vi "FRC Color Processing.vi"() -> ()   [LabVIEW 2017]
uses:
  <vilib>/Rock Robotics/WPI/Camera/WPI_CameraSettings Read MJPG.ctl
  <vilib>/Rock Robotics/WPI/Camera/WPI_CameraImageSize.ctl
  Vision Support Code/Camera Types.ctl
  <vilib>/Rock Robotics/WPI/Camera/WPI_CameraExposure Values.ctl
  <vilib>/Rock Robotics/WPI/Camera/WPI_CameraWhite Balance Values.ctl
  <vilib>/Rock Robotics/WPI/DriverStation/WPI_DriverStationAllianceInfo.ctl
  <vilib>/vision/NI_Vision_Development_Module.lvlib
panel:
  in  "Ring":u16(ring) items=["Cube", "Tape", "Switch LED", "Scale LED"]
  out "Angles":cluster{"Azimuth":dbl, "Elevation":dbl}[](array[cluster])
  in  "Vision Color Mode":u16(ring) items=["Alliance Color Range", "Reflective Tape", "Manual Color Range"]
  out "Game Specific Data":string
  out "Alliance":T1
  in  "Camera Address":string="USB 0"
  in  "Camera Settings":T2={"fps"=20, "compression"=30, "Image Size"=enum."320x240", "Config Shown"=FALSE}
  in  "Camera Settings 2":T6={"Exposure"=enum."Auto", "Exposure (%)"=50.0, "Brightness"=50, "White Balance"=enum."Auto", "Color Temp (K)"=0.0} {"Brightness" min=0 max=100}
  in  "Min Compnt %":dbl=15.0
  out "Results":T7(array[cluster]) {"Score" format="%#_3g"; "Pixels"."Rectangle"."Numeric 5" format="%#_3g"; "Pixels"."Rectangle"."Numeric 3" format="%#_3g"; "Pixels"."Rectangle"."Numeric 2" format="%#_3g"; "Pixels"."Rectangle"."Numeric" format="%#_3g"; "Normalized"."Rectangle"."Numeric 5" format="%#_2g"; "Normalized"."Rectangle"."Numeric 3" format="%#_2g"; "Normalized"."Rectangle"."Numeric 2" format="%#_2g"; "Normalized"."Rectangle"."Numeric" format="%#_2g"; "Normalized"."Center"."?" format="%#_3g"; "Normalized"."Center"."?" format="%#_3g"; "Distance (ft)" format="%#_3g"}
  in  "Size Limit %":dbl=0.04 min=0.0 max=100.0 step=0.01 format="%#_13g"
  out "Instructions:":string="Instructions:\nUse Source to load image files from a directory, or use a USB or IP camera connected to your laptop. Use Camera Settings 1 and 2 to achieve a dark image with bright and colorful stripes.\nLED Color can encoded as HSL or related color modes. Calibrate to the same color as the strips being reflected to the camera.\nClick and draw a line in Original Image to auto-calibrate the LED Color. You may want to widen and tweak Sat and Val by hand.\nThe Annotate button affects drawing a rectangle around the stripes and labeling it with a distance in ft. Distance relies on knowing the Camera Type and lens calibration (it looks up the lens view angle).\n\nAdjust Score Cutoff to make the code more or less picky. If the color is not very unique, you may need to increase the number of particles considered. The diagram uses a Size Limit to ignore colored things that are too small. You may need to adjust it if you are targetting from far away.\n\nResults give you the distance to the target, the center and box in a normalized (-1 to 1) and pixel coordinates.\n\nBe sure to read about setting camera exposure and brightness to help simplify your image and acquire color saturated images.\n\nThere are lots of comments on the diagram to explain the code."
  in  "Color Mode":u16(ring)=2 items=["RGB", "HSL", "HSV", "HSI"]
  in  "Particles":dbl=5.0
  in  "Score Cutoff %":dbl=75.0
  in  "Std Devs for Calibration":cluster{"H":dbl, "S":dbl, "V":dbl}={"H"=4.0, "S"=8.0, "V"=8.0}
  in  "Camera Type (for distance)":T8=enum."MS HD3000 square"
  in  "Annotate":bool=TRUE
  out "Qualified Particles":i32
  in  "LED Color Range":T9={"Hue"={75.46666717529297, 107.46666717529297}, "Sat"={221.18788146972656, 255.0}, "Val"={23.733230590820312, 172.13343811035156}} {"Hue" scale=0.0..255.0 scale format="%#_3g"}
  out "Mask":T10(plugin-control)
  out "Original Image":T10(plugin-control)
  # "Good target rectangle, distance ft"
  # "Bad target rectangle"
  # "Score in %"
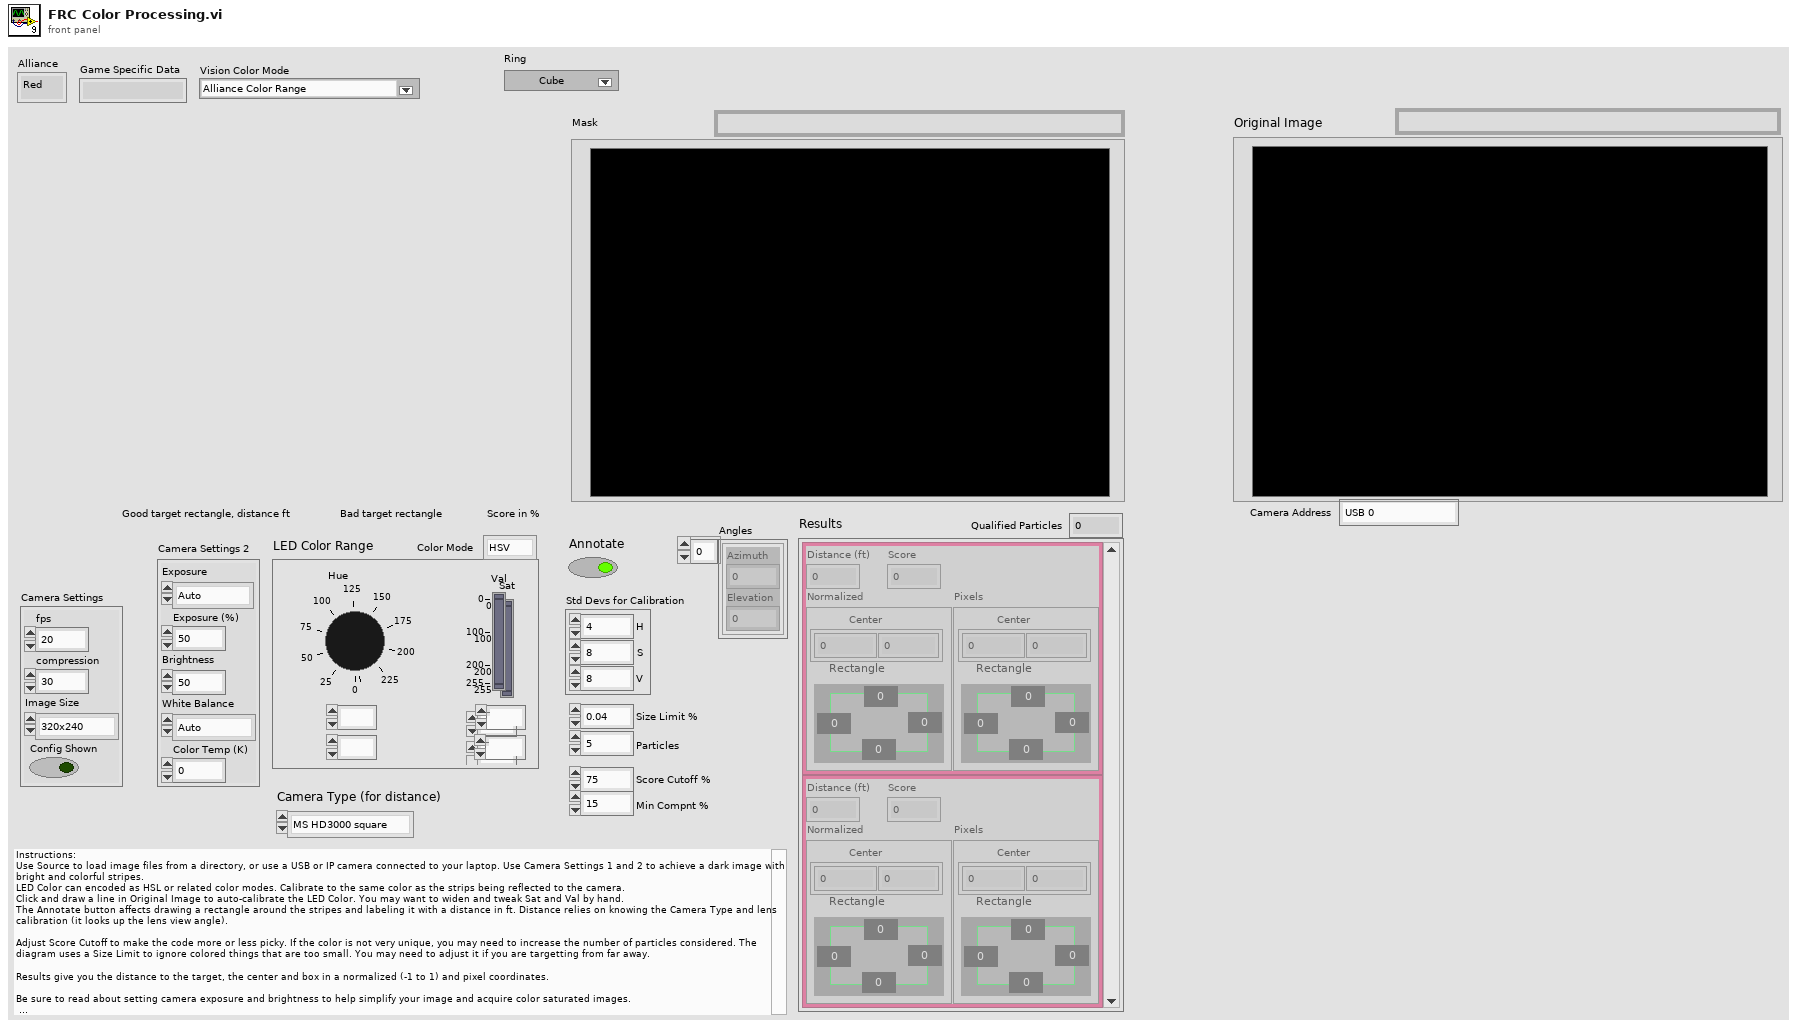
[diagram p1: front panel]
types:
  T1 = typedef "WPI_DriverStationAllianceInfo.ctl" = enum16{"Red", "Blue", "Invalid"}
  T2 = typedef "WPI_CameraSettings Read MJPG.ctl" = cluster{"fps":i32, "compression":i32, "Image Size":T3, "Config Shown":bool}
  T3 = typedef "WPI_CameraImageSize.ctl" = enum16{"640x480", "320x240", "160x120", "Custom"}
  T4 = typedef "WPI_CameraExposure Values.ctl" = enum16{"Auto", "Flicker-free 50 Hz", "Flicker-free 60 Hz", "Hold current", "Custom"}
  T5 = typedef "WPI_CameraWhite Balance Values.ctl" = enum16{"Auto", "Fixed indoor", "Fixed outdoor 1", "Fixed outdoor 2", "Fixed fluorescent 1", "Fixed fluorescent 2", "Hold current", "Custom"}
  T6 = cluster{"Exposure":T4, "Exposure (%)":dbl, "Brightness":i32, "White Balance":T5, "Color Temp (K)":dbl}
  T7 = cluster{"Distance (ft)":dbl, "Score":dbl, "Normalized":cluster{"Center":cluster{dbl, dbl}, "Rectangle":cluster{"Numeric":dbl, "Numeric 2":dbl, "Numeric 3":dbl, "Numeric 5":dbl}}, "Pixels":cluster{"Center":cluster{dbl, dbl}, "Rectangle":cluster{"Numeric":dbl, "Numeric 2":dbl, "Numeric 3":dbl, "Numeric 5":dbl}}}[]
  T8 = typedef "Camera Types.ctl" = enum16{"206", "1011", "1013", "MS HD3000 square", "MS HD3000 640x480"}
  T9 = cluster{"Hue":cluster{dbl, dbl}, "Sat":cluster{dbl, dbl}, "Val":cluster{dbl, dbl}}
  T10 = typedef "IMAQ Image.ctl" = refnum<image>
  T11 = typedef "Particle Parameters" = i32
  T12 = typedef "Image Type" = u32
  T13 = enum8{"Enabled", "Disabled", "Disabled and Grayed Out"}
  T14 = cluster{cluster{dbl, dbl}, cluster{dbl, dbl}, cluster{dbl, dbl}}
  T15 = cluster{"Score":dbl, "Rect":cluster{"Left":dbl, "Top":dbl, "Right":dbl, "Bottom":dbl}, "Full Scores":cluster{"Aspect Ratio":dbl, "Top Position":dbl, "Bottom Position":dbl, "Left Gap":dbl, "Width":dbl, "Height Ratio":dbl}}[]
  T16 = cluster{"Left":dbl, "Top":dbl, "Right":dbl, "Bottom":dbl}
  T17 = cluster{"Distance (ft)":dbl, "Score":dbl, "Normalized":cluster{"Center":cluster{dbl, dbl}, "Rectangle":cluster{"Numeric":dbl, "Numeric 2":dbl, "Numeric 3":dbl, "Numeric 5":dbl}}, "Pixels":cluster{"Center":cluster{dbl, dbl}, "Rectangle":cluster{"Numeric":dbl, "Numeric 2":dbl, "Numeric 3":dbl, "Numeric 5":dbl}}}
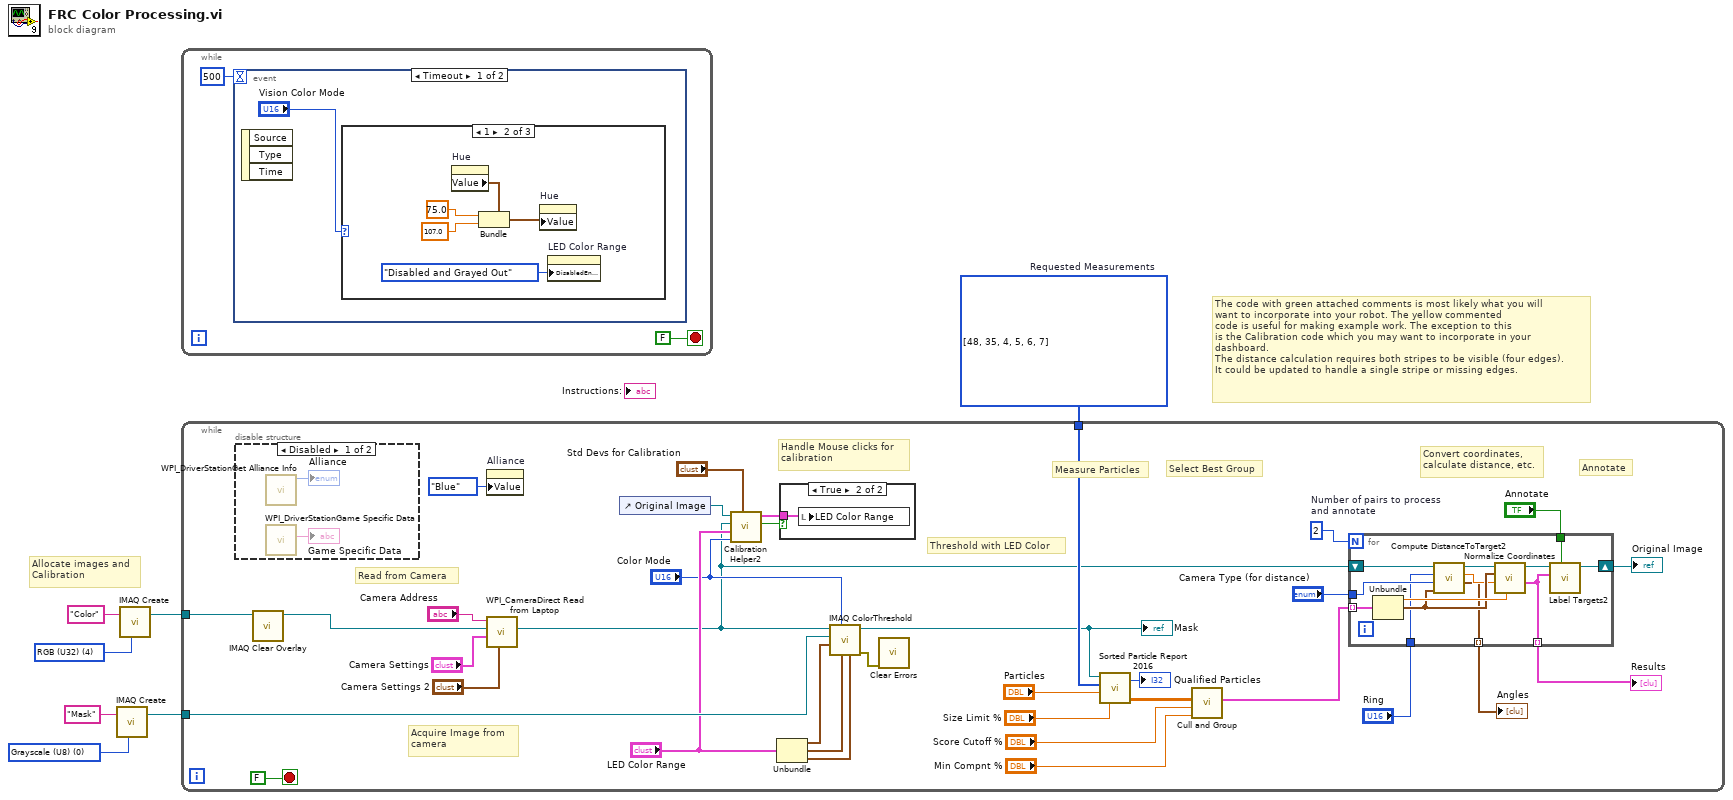
[diagram p0: block diagram]
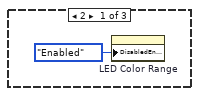
[diagram p2: hidden frame]
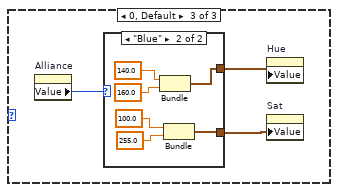
[diagram p3: hidden frame]
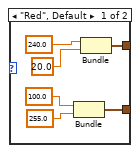
[diagram p4: hidden frame]
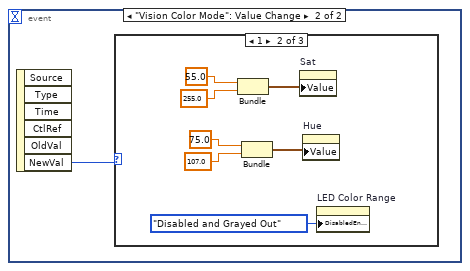
[diagram p5: hidden frame]
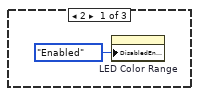
[diagram p6: hidden frame]
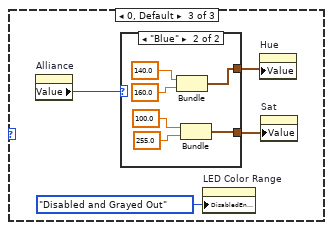
[diagram p7: hidden frame]
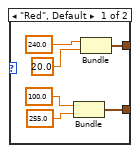
[diagram p8: hidden frame]
diagram:
  w2 = T11[] [48, 35, 4, 5, 6, 7] items=["Center of Mass X", "Center of Mass Y", "First Pixel X", "First Pixel Y", "Bounding Rect Left", "Bounding Rect Top", "Bounding Rect Right", "Bounding Rect Bottom", "Max Feret Diameter Start X", "Max Feret Diameter Start Y", "Max Feret Diameter End X", "Max Feret Diameter End Y", "Max Horiz. Segment Length Left", "Max Horiz. Segment Length Right", "Max Horiz. Segment Length Row", "-", "Bounding Rect Width", "Bounding Rect Height", "Bounding Rect Diagonal", "Perimeter", "Convex Hull Perimeter", "Holes' Perimeter", "Max Feret Diameter", "Equivalent Ellipse Major Axis", "Equivalent Ellipse Minor Axis", "Equivalent Ellipse Minor Axis (Feret)", "Equivalent Rect Long Side", "Equivalent Rect Short Side", "Equivalent Rect Diagonal", "Equivalent Rect Short Side (Feret)", "Average Horiz. Segment Length", "Average Vert. Segment Length", "Hydraulic Radius", "Waddel Disk Diameter", "-", "Area", "Holes' Area", "Particle & Holes' Area", "Convex Hull Area", "Image Area", "-", "Number of Holes", "Number of Horiz. Segments", "Number of Vert. Segments", "-", "Orientation", "Max Feret Diameter Orientation", "-", "% Area/Image Area", "% Area/(Particle & Holes' Area)", "Ratio of Equivalent Ellipse Axes", "Ratio of Equivalent Rect Sides", "-", "Elongation Factor", "Compactness Factor", "Heywood Circularity Factor", "Type Factor", "-", "Sum X", "Sum Y", "Sum XX", "Sum XY", "Sum YY", "Sum XXX", "Sum XXY", "Sum XYY", "Sum YYY", "-", "Moment of Inertia XX", "Moment of Inertia XY", "Moment of Inertia YY", "Moment of Inertia XXX", "Moment of Inertia XXY", "Moment of Inertia XYY", "Moment of Inertia YYY", "Norm. Moment of Inertia XX", "Norm. Moment of Inertia XY", "Norm. Moment of Inertia YY", "Norm. Moment of Inertia XXX", "Norm. Moment of Inertia XXY", "Norm. Moment of Inertia XYY", "Norm. Moment of Inertia YYY", "Hu Moment 1", "Hu Moment 2", "Hu Moment 3", "Hu Moment 4", "Hu Moment 5", "Hu Moment 6", "Hu Moment 7"]  # Requested Measurements
  w5 = T12 0 items=["Grayscale (U8)", "Grayscale (I16)", "Grayscale (SGL)", "Complex (CSG)", "RGB (U32)", "HSL (U32)", "RGB (U64)", "Grayscale (U16)"] ("Image Type")
  w6 = T12 4 items=["Grayscale (U8)", "Grayscale (I16)", "Grayscale (SGL)", "Complex (CSG)", "RGB (U32)", "HSL (U32)", "RGB (U64)", "Grayscale (U16)"] ("Image Type")
  # "The code with green attached comments is most likely what you will\nwant to incorporate into your robot. The yellow commented\ncode is useful for making example work. The exception to this\nis the Calibration code which you may want to incorporate in your\ndashboard.\nThe distance calculation requires both stripes to be visible (four edges).\nIt could be updated to handle a single stripe or missing edges."
  # "Allocate images and\nCalibration"
  n1 = call "IMAQ Create"("Image Name"="Mask", "Image Type"=w5) -> ("New Image"=w3:T10)  [unwired: 2 in, 2 out]
  n2 = call "IMAQ Create"("Image Name"="Color", "Image Type"=w6) -> ("New Image"=w1:T10)  [unwired: 2 in, 2 out]
  n3 = while {
    stop <- FALSE stop-if-true
    n4 = event shown="[0] Timeout" {
      selector: _ -> [_ _]
      dyn-events: _ -> [_ _]
      timeout: 500 -> [_ _]
      event Timeout {
        n5 = event-data() -> ()  [unwired: 1 in, 3 out]
        n6 = case shown="1" "Vision Color Mode" {
          frame 2 {
            n7 = property on="LED Color Range" class="Clust (strict)"("DisabledEnum"=T13."Enabled" ("Disabled")) -> ()  [unwired: 2 in, 2 out]
          }
          frame 1 {
            n8 = property on="Hue" class="Knob (strict)"() -> ("Value"=w16:cluster{dbl, dbl})  [unwired: 2 in, 2 out]
            n9 = Bundle(cluster=w16, 75.0, 107.0) -> (w15:cluster{dbl, dbl})
            n10 = property on="Hue" class="Knob (strict)"("Value"=w15) -> ()  [unwired: 2 in, 2 out]
            n11 = property on="LED Color Range" class="Clust (strict)"("DisabledEnum"=T13."Disabled and Grayed Out" ("Disabled")) -> ()  [unwired: 2 in, 2 out]
          }
          frame 0, Default {
            n12 = property on="Alliance" class="Enum (strict)"() -> ("Value"=w17:T1)  [unwired: 2 in, 2 out]
            n13 = case shown="\"Blue\"" w17 {
              tunnel: [w21 w27] -> w19
              tunnel: [w20 w26] -> w18
              frame "Red", Default {
                n14 = Bundle(100.0, 255.0) -> (w20:cluster{dbl, dbl})  [unwired: 1 in]
                n15 = Bundle(240.0, 20.0) -> (w21:cluster{dbl, dbl})  [unwired: 1 in]
              }
              frame "Blue" {
                n16 = Bundle(140.0, 160.0) -> (w27:cluster{dbl, dbl})  [unwired: 1 in]
                n17 = Bundle(100.0, 255.0) -> (w26:cluster{dbl, dbl})  [unwired: 1 in]
              }
            }
            n18 = property on="Hue" class="Knob (strict)"("Value"=w19) -> ()  [unwired: 2 in, 2 out]
            n19 = property on="Sat" class="Slide (strict)"("Value"=w18) -> ()  [unwired: 2 in, 2 out]
          }
        }
      }
      event "Vision Color Mode": Value Change {
        n20 = event-data() -> ("NewVal"=w32:u16)  [unwired: 1 in, 5 out]
        n21 = case shown="1" w32 {
          frame 2 {
            n22 = property on="LED Color Range" class="Clust (strict)"("DisabledEnum"=T13."Enabled" ("Disabled")) -> ()  [unwired: 2 in, 2 out]
          }
          frame 1 {
            n23 = Bundle(55.0, 255.0) -> (w34:cluster{dbl, dbl})  [unwired: 1 in]
            n24 = Bundle(75.0, 107.0) -> (w39:cluster{dbl, dbl})  [unwired: 1 in]
            n25 = property on="Sat" class="Slide (strict)"("Value"=w34) -> ()  [unwired: 2 in, 2 out]
            n26 = property on="Hue" class="Knob (strict)"("Value"=w39) -> ()  [unwired: 2 in, 2 out]
            n27 = property on="LED Color Range" class="Clust (strict)"("DisabledEnum"=T13."Disabled and Grayed Out" ("Disabled")) -> ()  [unwired: 2 in, 2 out]
          }
          frame 0, Default {
            n28 = property on="Alliance" class="Enum (strict)"() -> ("Value"=w41:T1)  [unwired: 2 in, 2 out]
            n29 = case shown="\"Blue\"" w41 {
              tunnel: [w46 w52] -> w43
              tunnel: [w45 w51] -> w42
              frame "Red", Default {
                n30 = Bundle(100.0, 255.0) -> (w45:cluster{dbl, dbl})  [unwired: 1 in]
                n31 = Bundle(240.0, 20.0) -> (w46:cluster{dbl, dbl})  [unwired: 1 in]
              }
              frame "Blue" {
                n32 = Bundle(140.0, 160.0) -> (w52:cluster{dbl, dbl})  [unwired: 1 in]
                n33 = Bundle(100.0, 255.0) -> (w51:cluster{dbl, dbl})  [unwired: 1 in]
              }
            }
            n34 = property on="LED Color Range" class="Clust (strict)"("DisabledEnum"=T13."Disabled and Grayed Out" ("Disabled")) -> ()  [unwired: 2 in, 2 out]
            n35 = property on="Hue" class="Knob (strict)"("Value"=w43) -> ()  [unwired: 2 in, 2 out]
            n36 = property on="Sat" class="Slide (strict)"("Value"=w42) -> ()  [unwired: 2 in, 2 out]
          }
        }
      }
    }
  }
  n37 = while {
    tunnel: w1 -> [w66]
    tunnel: w3 -> [w90]
    tunnel: w2 -> [w86]
    stop <- FALSE stop-if-true
    w68 = 2  # Number of pairs to process and annotate
    # "Read from Camera"
    # "Handle Mouse clicks for\ncalibration"
    # "Measure Particles"
    # "Convert coordinates,\ncalculate distance, etc."
    # "Annotate"
    # "Select Best Group"
    # "Threshold with LED Color"
    # "Acquire Image from\ncamera"
    n38 = disable-structure shown="Disabled" {
      frame Disabled {
        n39 = call <vilib>:"WPI_DriverStationGet Alliance Info.vi"() -> ("Alliance"=→"Alliance":T1)  [unwired: 6 in, 5 out]
        n40 = call <vilib>:"WPI_DriverStationGame Specific Data.vi"() -> ("Game Specific Data"=→"Game Specific Data":string)  [unwired: 11 in]
      }
      frame Enabled {
      }
    }
    n41 = call "IMAQ Clear Overlay"("Image"=w66) -> ("Image Out"=w65:T10)  [unwired: 2 in, 8 out]
    n42 = property on="Alliance" class="Enum (strict)"("Value"=WPI_DriverStationAllianceInfo."Blue" ("Alliance")) -> ()  [unwired: 2 in, 2 out]
    n43 = call <vilib>:"WPI_CameraDirect Read from Laptop.vi"("Camera Settings 2"="Camera Settings 2", "Camera Settings"="Camera Settings", "Image"=w65, "address"="Camera Address") -> ("Image Out"=w67:T10)  [unwired: 6 in, 1 out]
    n44 = control-ref of="Original Image"() -> (w82:refnum<vi>)
    n45 = call "Calibration Helper2.vi"("Std Devs"="Std Devs for Calibration", "Color Mode"="Color Mode", "Color Components"="LED Color Range", "Image"=w67, "Image Ctl Refnum"=w82) -> ("Changed"=w81:bool, "output color"=w80:T14)  [unwired: 5 in]
    n46 = Unbundle("LED Color Range") -> ("Hue"=w89:cluster{dbl, dbl}, "Sat"=w88:cluster{dbl, dbl}, "Val"=w87:cluster{dbl, dbl})
    n47 = case shown="True" w81 {
      tunnel: w80 -> [_ w107]
      frame False {
      }
      frame True {
        n48 = local write "LED Color Range"(w107) -> ()
      }
    }
    n49 = call "IMAQ ColorThreshold"("Blue or Luma or Val or Inten Range"=w87, "Green or Sat Range"=w88, "Color Mode"="Color Mode", "Red or Hue Range"=w89, "Image Dst"=w90, "Image Src"=w67) -> ("error out"=w83:errorcluster, "Image Dst Out"=w76:T10)  [unwired: 4 in]
    "Mask" <- w76
    n50 = call <vilib>:"Clear Errors.vi"("error in (no error)"=w83) -> ()  [unwired: 5 in, 2 out]
    n51 = call "Sorted Particle Report 2016.vi"("Min Area Size %"="Size Limit %", "Particle Count Limit"="Particles", "Pixel Measurements"=w86, "Image in"=w76) -> ("Sorted Data"=w77:dbl[][], "Particles"=→"Qualified Particles":i32)
    n52 = call "Cull and Group.vi"("Min Compnt %"="Min Compnt %", "Score Cutoff %"="Score Cutoff %", "Sorted Data"=w77) -> ("Best Targets above cutoff"=w75:T15)  [unwired: 8 in]
    n53 = for {
      N: w68 -> [_]
      tunnel: [w105] -> w64 mode=indexing
      tunnel: w75 -> [w101] mode=indexing
      tunnel: "Camera Type (for distance)" -> [w104]
      tunnel: "Annotate" -> [w97]
      shift-right: [w102] -> w69
      shift-left: w67 -> [w103]
      tunnel: [w95] -> w58 mode=indexing
      tunnel: "Ring" -> [w94]
      n54 = Unbundle(w101) -> ("Score"=w100:dbl, "Rect"=w98:T16)  [unwired: 1 out]
      n55 = call "Compute DistanceToTarget2.vi"("Rect"=w98, "Camera Type"=w104, "Ring"=w94, "Image Src"=w103) -> ("Angles"=w95:cluster{"Azimuth":dbl, "Elevation":dbl}, "Distance (ft)"=w96:dbl, "Image Dst Out"=w99:T10)  [unwired: 5 in]
      n56 = call "Normalize Coordinates.vi"("Score"=w100, "Distance"=w96, "Bounding box"=w98, "Image in"=w99) -> ("Results"=w105:T17, "Image out"=w106:T10)  [unwired: 6 in]
      n57 = call "Label Targets2.vi"("Annotate"=w97, "Results"=w105, "Image in"=w106) -> ("Image out"=w102:T10)  [unwired: 8 in]
    }
    "Original Image" <- w69
    "Results" <- w64
    "Angles" <- w58
  }
